vi "Fit Result to String.vi"(8 "error in (no error)":errorcluster, 11 "Head Impulse Fit in":refnum<class "Head Impulse Fit.lvclass">) -> (0 "error out":errorcluster, 2 "Array":string[](array[string]), 3 "Head Impulse Fit out":refnum<class "Head Impulse Fit.lvclass">)   [LabVIEW 2014, in "Head Impulse Fit.lvclass"]
uses:
  Head Impulse Fit.lvclass
  Head Impulse Fit.lvclass/Head Impulse Fit.ctl
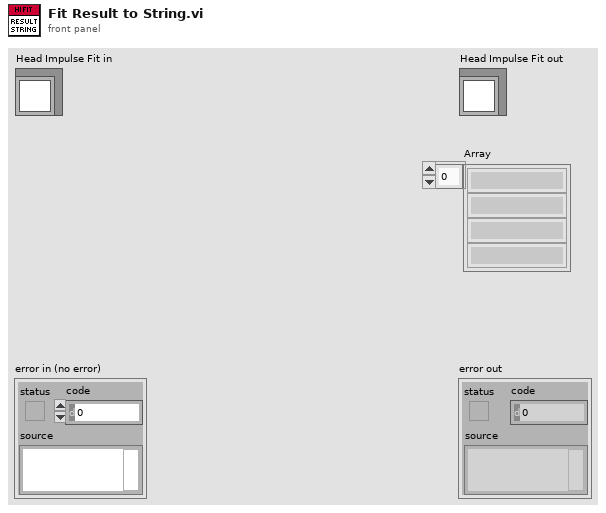
[diagram p1: front panel]
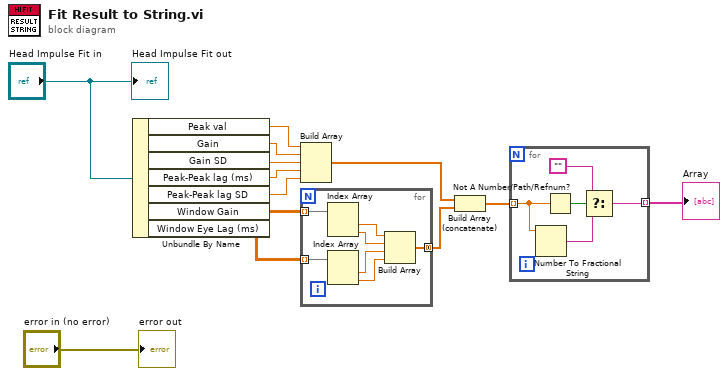
[diagram p0: block diagram]
diagram:
  n1 = Unbundle By Name("Head Impulse Fit in") -> ("Peak val"=w1:dbl, "Gain"=w11:dbl, "Gain SD"=w10:dbl, "Peak-Peak lag (ms)"=w9:dbl, "Peak-Peak lag SD"=w8:dbl, "Window Gain"=w7:dbl[][], "Window Eye Lag (ms)"=w6:dbl[][])
  n2 = Build Array(w1, w11, w10, w9, w8) -> (w4:dbl[])
  n3 = for {
    tunnel: w7 -> [w20] mode=indexing
    tunnel: w6 -> [w19] mode=indexing
    tunnel: [w14] -> w5 mode=concatenating
    n4 = Index Array(array=w20) -> (element #1=w18:dbl, element #2=w17:dbl)  [unwired: 2 in]
    n5 = Index Array(array=w19) -> (element #1=w16:dbl, element #2=w15:dbl)  [unwired: 2 in]
    n6 = Build Array(w18, w17, w16, w15) -> (w14:dbl[])
  }
  n7 = Build Array (concatenate)(w4, w5) -> (w3:dbl[])
  n8 = for {
    tunnel: [w25] -> w2 mode=indexing
    tunnel: w3 -> [w21] mode=indexing
    n9 = Number To Fractional String(number=w21) -> (F-format string=w22:string)  [unwired: 3 in]
    n10 = Not A Number/Path/Refnum?(number/path/refnum=w21) -> (NaN/Path/Refnum?=w24:bool)
    n11 = Select(t="", s=w24, f=w22) -> (s? t:f=w25:string)
  }
  "Array" <- w2
  "error out" <- "error in (no error)"
  "Head Impulse Fit out" <- "Head Impulse Fit in"
